vi "ief_connnect_2_SV_u32.vi"(8 "error in (no error)":errorcluster, 11 "shared variable refnum in":string) -> (0 "error out":errorcluster, 3 "Variable Name Control/Indicator":refnum<k21>)   [LabVIEW 2015, in "IEF Werner.lvlib"]
uses:
  IEF Werner.lvlib
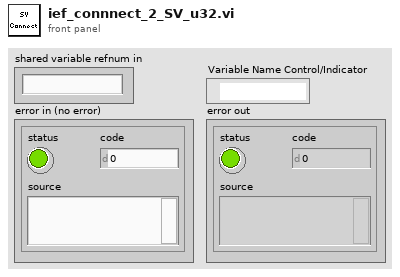
[diagram p1: front panel]
types:
  T1 = cluster{"Read Access":enum8{"Allowed", "Required", "None"}, "Write Access":enum8{"Allowed", "Required", "None"}}
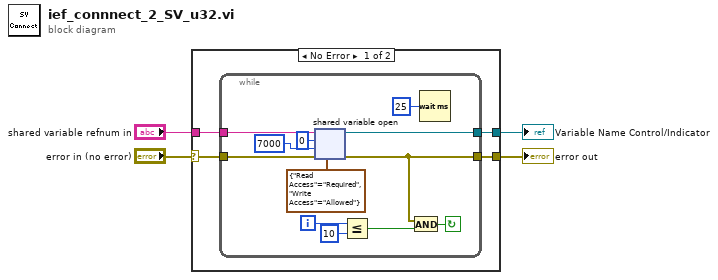
[diagram p0: block diagram]
diagram:
  n1 = case shown="No Error" "error in (no error)" {
    selector: "error in (no error)" -> [w6 w21]
    tunnel: "shared variable refnum in" -> [w8 _]
    tunnel: [w7 _] -> w1
    tunnel: [w5 w21] -> w2
    frame No Error {
      n2 = while {
        tunnel: w8 -> [w18]
        tunnel: [w17] -> w7
        tunnel: w6 -> [w16]
        tunnel: [w12] -> w5
        i -> [w14]
        stop <- w10 continue-if-true
        n3 = shared-variable-open(w18, w16, u32 0 ("data type"), T1 {"Read Access"=enum."Required", "Write Access"=enum."Allowed"} ("access"), 7000 ("timeout ms")) -> (w17:refnum<k21>, w12:errorcluster)  [unwired: 1 in]
        n4 = Less Or Equal?(x=w14, y=10) -> (x <= y?=w11:bool)
        n5 = And(x=w12, y=w11) -> (x .and. y?=w10:bool)
        n6 = Wait (ms)(milliseconds to wait=u32 25) -> ()  [unwired: 1 out]
      }
    }
    frame Error {
    }
  }
  "error out" <- w2
  "Variable Name Control/Indicator" <- w1
